vi "Initialize Display.vi"(8 "Error In":errorcluster, 11 "Dashboard In":refnum<class "Dashboard.lvclass">) -> (0 "Error Out":errorcluster, 3 "Dashboard Out":refnum<class "Dashboard.lvclass">)   [LabVIEW 2019, in "Dashboard.lvclass"]
uses:
  Dashboard.lvclass
  <vilib>/Memosfet/myRIO-Neopixel/RT/Display Utilities/Public/Controls/2D Dimensions.ctl
  Accessors/Display/Set Display.vi
  Accessors/Processes/Get Processes.vi
  Draw Frame/Accessors/Display/Set Display.vi
  Display Manager/Accessors/Display/Set Display.vi
  Display Manager/Display Manager.lvclass
  Audio Analyzer/Audio Analyzer.lvclass
  Draw Frame/Draw Frame.lvclass
  Error Handling/Error Handling.lvclass
  Sequencer/Sequencer.lvclass
  <vilib>/Memosfet/myRIO-Neopixel/RT/Display Utilities/Display Utilities.lvlib
  <vilib>/Memosfet/myRIO-Neopixel/RT/Display/Display.lvclass
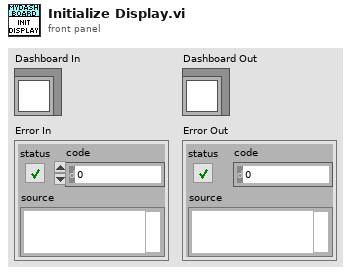
[diagram p1: front panel]
types:
  T1 = typedef "Display Utilities.lvlib/2D Dimensions.ctl" = cluster{"Width":i32, "Height":i32}
  T2 = typedef "Dashboard.lvclass/Processes.ctl" = cluster{"Display Manager":refnum<class "Display Manager.lvclass">, "Audio Analyzer":refnum<class "Audio Analyzer.lvclass">, "Draw Frame":refnum<class "Draw Frame.lvclass">, "Error Handling":refnum<class "Error Handling.lvclass">, "Sequencer":refnum<class "Sequencer.lvclass">}
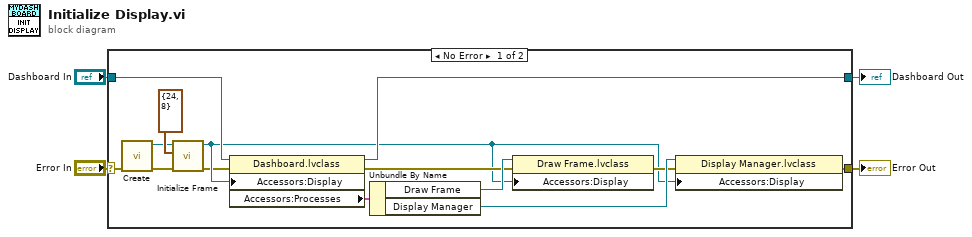
[diagram p0: block diagram]
diagram:
  n1 = case shown="No Error" "Error In" {
    selector: "Error In" -> [w7 w20]
    tunnel: [w11 w20] -> w4
    tunnel: [w18 w19] -> w3
    tunnel: "Dashboard In" -> [w17 w19]
    frame No Error {
      n2 = call <vilib>:"Create.vi"("Error In"=w7) -> ("Error Out"=w8:errorcluster, "Screen Out"=w9:refnum<class "Display.lvclass">)  [unwired: 9 in]
      n3 = call <vilib>:"Initialize Frame.vi"("Error In"=w8, "Size"=T1 {"Width"=24, "Height"=8}, "Display In"=w9) -> ("Error Out"=w5:errorcluster, "Display Out"=w6:refnum<class "Display.lvclass">)  [unwired: 7 in]
      n4 = property class="Dashboard.lvclass"(reference=w17, error in=w5, "Accessors:Display"=w6) -> (reference out=w18:refnum<class "Dashboard.lvclass">, error out=w13:errorcluster, "Accessors:Processes"=w16:T2)
      n5 = Unbundle By Name(w16) -> ("Draw Frame"=w15:refnum<class "Draw Frame.lvclass">, "Display Manager"=w14:refnum<class "Display Manager.lvclass">)
      n6 = property class="Draw Frame.lvclass"(reference=w15, error in=w13, "Accessors:Display"=w6) -> (error out=w12:errorcluster)  [unwired: 1 out]
      n7 = property class="Display Manager.lvclass"(reference=w14, error in=w12, "Accessors:Display"=w6) -> (error out=w11:errorcluster)  [unwired: 1 out]
    }
    frame Error {
    }
  }
  "Error Out" <- w4
  "Dashboard Out" <- w3
